vi "Scan DQMH Modules.vi"(11 "error in":errorcluster) -> (4 "DQMH Modules":refnum<vi>[](array[refnum]), 6 "Modules List":string[](array[string]), 8 "Module Description":string[](array[string]), 10 "Cloneable?":bool[](array[boolean]), 15 "error out":errorcluster)   [LabVIEW 2020, in "Panther Dashboard.lvlib"]
doc: "Gets the Singleton and Cloneable references and creates a list of each type of DQMH Modules"
uses:
  Panther Dashboard.lvlib
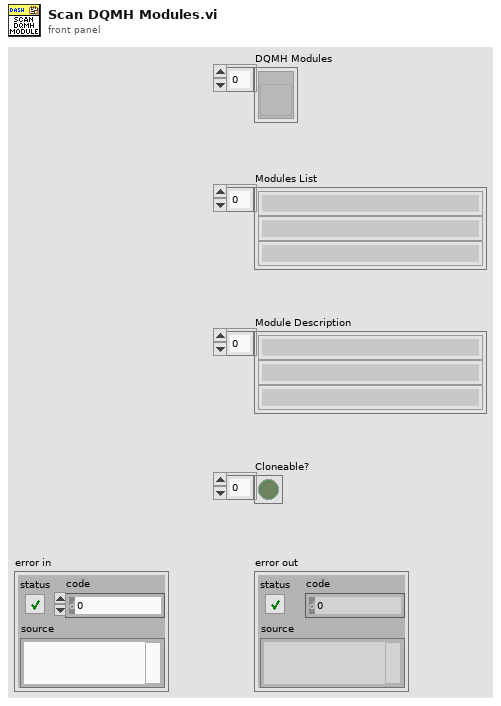
[diagram p1: front panel]
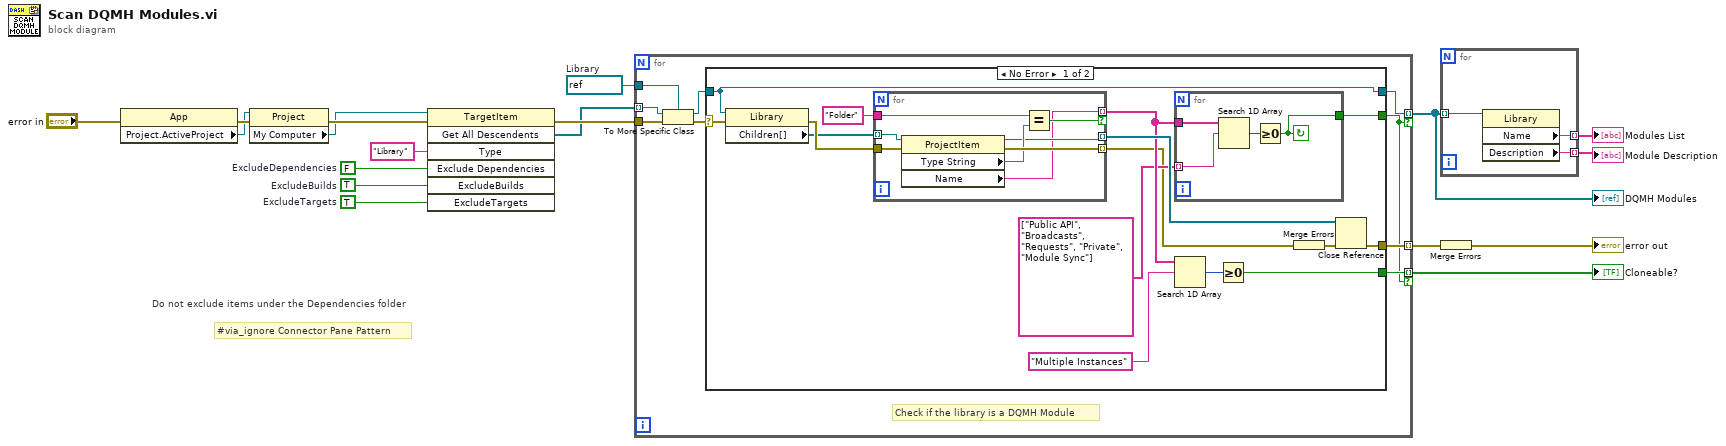
[diagram p0: block diagram]
diagram:
  w7 = refnum<vi> refnum  # Library
  w8 = FALSE  # ExcludeDependencies
  w9 = TRUE  # ExcludeTargets
  w10 = TRUE  # ExcludeBuilds
  # "#via_ignore Connector Pane Pattern"
  # "Do not exclude items under the Dependencies folder"
  n1 = property class="App"(error in="error in") -> (error out=w16:errorcluster, "Project.ActiveProject"=w12:refnum<vi>)  [unwired: 1 in, 1 out]
  n2 = property class="Project"(reference=w12, error in=w16) -> (error out=w17:errorcluster, "My Computer"=w11:refnum<vi>)  [unwired: 1 out]
  n3 = invoke class="TargetItem" method="Get All Descendents"(reference=w11, error in=w17, "Type"="Library", "Exclude Dependencies"=w8, "ExcludeBuilds"=w10, "ExcludeTargets"=w9) -> (error out=w18:errorcluster, "All Descendents"=w6:refnum<vi>[])  [unwired: 1 in, 5 out]
  n4 = for {
    tunnel: w7 -> [w24]
    tunnel: [w23] -> w3 mode=indexing if=w19
    tunnel: w6 -> [w21] mode=indexing
    tunnel: [w26] -> w5 mode=indexing
    tunnel: w18 -> [w25]
    tunnel: [w20] -> w2 mode=indexing if=w19
    # "Check if the library is a DQMH Module"
    n5 = To More Specific Class(target class=w24, reference=w21, error in=w25) -> (specific class reference=w22:refnum<vi>, error out=w27:errorcluster)
    n6 = case shown="No Error" w27 {
      selector: w27 -> [w42 _]
      tunnel: w22 -> [w37 _]
      tunnel: [w38 _] -> w19
      tunnel: [w37 _] -> w23
      tunnel: [w41 _] -> w26
      tunnel: [w36 _] -> w20
      frame No Error {
        n7 = property class="Library"(reference=w37, error in=w42) -> (error out=w40:errorcluster, "Children[]"=w34:refnum<vi>[])  [unwired: 1 out]
        n8 = for {
          tunnel: [w47] -> w30 mode=indexing if=w48
          tunnel: w40 -> [w54]
          tunnel: [w53] -> w28 mode=indexing
          tunnel: [w50] -> w33 mode=indexing
          tunnel: w34 -> [w52] mode=indexing
          tunnel: "Folder" ("Type") -> [w49]
          n9 = property class="ProjectItem"(reference=w52, error in=w54) -> (reference out=w50:refnum<vi>, error out=w53:errorcluster, "Type String"=w51:string, "Name"=w47:string)
          n10 = Equal?(x=w49, y=w51) -> (x = y?=w48:bool)
        }
        n11 = for {
          tunnel: string[] ["Public API", "Broadcasts", "Requests", "Private", "Module Sync"] -> [w46] mode=indexing
          tunnel: w30 -> [w45]
          tunnel: [w43] -> w38
          stop <- w43 continue-if-true
          n12 = Search 1D Array(1D array=w45, element=w46) -> (index of element=w44:i32)  [unwired: 1 in]
          n13 = Greater Or Equal To 0?(x=w44) -> (x >= 0?=w43:bool)
        }
        n14 = Search 1D Array(1D array=w30, element="Multiple Instances") -> (index of element=w32:i32)  [unwired: 1 in]
        n15 = Greater Or Equal To 0?(x=w32) -> (x >= 0?=w36:bool)
        n16 = Merge Errors(w28) -> (w39:errorcluster)
        n17 = Close Reference(reference=w33, error in (no error)=w39) -> (error out=w41:errorcluster)
      }
      frame Error {
      }
    }
  }
  "DQMH Modules" <- w3
  "Cloneable?" <- w2
  n18 = for {
    tunnel: [w57] -> w13 mode=indexing
    tunnel: w3 -> [w56] mode=indexing
    tunnel: [w55] -> w1 mode=indexing
    n19 = property class="Library"(reference=w56) -> ("Name"=w57:string, "Description"=w55:string)  [unwired: 1 in, 2 out]
  }
  "Modules List" <- w13
  "Module Description" <- w1
  n20 = Merge Errors(w5) -> (→"error out":errorcluster)
